vi "XNET_Frame_InStream_Read.vi"() -> ()   [LabVIEW 2018]
uses:
  <vilib>/xnet/xnet.llb/XNET Frame CAN.ctl
  <vilib>/xnet/xnet.llb/XNET Frame Type CAN.ctl
  <vilib>/xnet/xnet.llb/XNET Read (Frame CAN).vi
  <vilib>/xnet/xnet.llb/XNET Create Session (Frame Input Stream).vi
  <resource>/objmgr/xnet.rc
panel:
  out "data 2":T1[](array[typedef]) {"payload" format="%x"; "timestamp" format="%<%.7X\n%x>T"; "type" items=["CAN Data"=0, "CAN Remote"=1, "CAN Bus Error"=2, "CAN 2.0 Data"=8, "CAN FD Data"=16, "CAN FD+BRS Data"=24, "J1939 Data"=192, "Delay"=224, "Log Trigger"=225, "Start Trigger"=226]; "identifier" format="%x"}
  in  "Boolean":bool
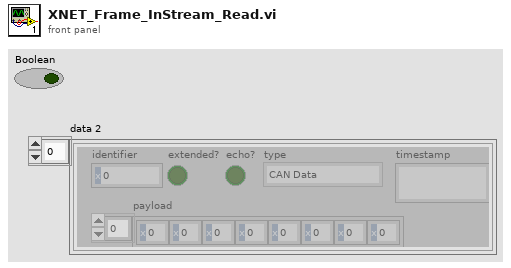
[diagram p1: front panel]
types:
  T1 = typedef "XNET Frame CAN.ctl" = cluster{"timestamp":timestamp, "payload":u8[], "identifier":u32, "type":T2, "extended?":bool, "echo?":bool}
  T2 = typedef "XNET Frame Type CAN.ctl" = u8
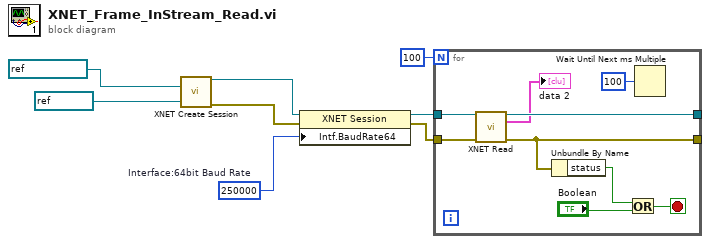
[diagram p0: block diagram]
diagram:
  w6 = u64 250000  # Interface:64bit Baud Rate
  n1 = call-poly <vilib>:"XNET Create Session.vi"("cluster (:memory:)"=refnum<k21> ":memory:", "interface"=refnum<k21> "CAN1") -> ("session out"=w7:refnum<k21>, "error out"=w4:errorcluster)  [unwired: 12 in]
  n2 = property class="XNET Session"(reference=w7, error in=w4, "Intf.BaudRate64"=w6) -> (reference out=w3:refnum<k21>, error out=w2:errorcluster)
  n3 = for {
    N: 100 -> [_]
    tunnel: w3 -> [w17]
    tunnel: w2 -> [w16]
    tunnel: [w15] -> _
    tunnel: [w14] -> _
    stop <- w13 stop-if-true
    n4 = call-poly <vilib>:"XNET Read.vi"("session in"=w17, "error in (no error)"=w16) -> ("session out"=w15:refnum<k21>, "data"=→"data 2":T1[], "error out"=w14:errorcluster)  [unwired: 10 in, 1 out]
    n5 = Unbundle By Name(w14) -> ("status"=w12:bool)
    n6 = Or(x=w12, y="Boolean") -> (x .or. y?=w13:bool)
    n7 = Wait Until Next ms Multiple(millisecond multiple=u32 100) -> ()  [unwired: 1 out]
  }
